vi "Y to D Conversion (Waveform).vi"(0 "phase voltage waveforms":waveform(dbl)[](array[waveform]), 9 "system info in":refnum<class "EP System Info.lvclass">, 11 "error in (no error)":errorcluster) -> (4 "line voltage waveforms":waveform(dbl)[](array[waveform]), 10 "system info out":refnum<class "EP System Info.lvclass">, 15 "error out":errorcluster)   [LabVIEW 2014, in "NI_EP_Power Quality.lvlib"]
doc: "Converts phase voltages to line voltages. You must manually select the polymorphic instance you want to use.\n\nThis VI supports measuring single-line and multiple-line systems."
uses:
  <vilib>/addons/Electrical Power/PQ/NI_EP_Power Quality.lvlib
  <vilib>/addons/Electrical Power/PQ/Common/Classes/System Info/EP System Info.lvclass
  <vilib>/addons/Electrical Power/Motor Monitoring/NI_EP_Motor Monitoring.lvlib
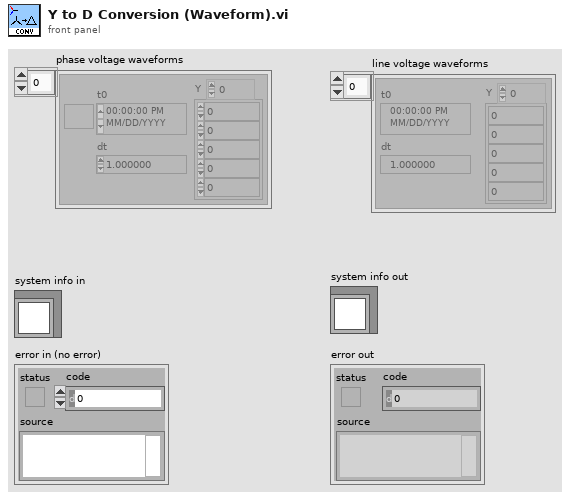
[diagram p1: front panel]
types:
  T1 = typedef "NI_EP_Power Quality.lvlib/ep_Wiring.ctl" = enum16{"4xUph + 4xI", "3xUph + 4xI", "3xUline + 4xI", "3xUph + 3xI", "3xUline + 3xI", "3xUph + 2xI", "3xUline + 2xI", "1xUph + 1xI"}
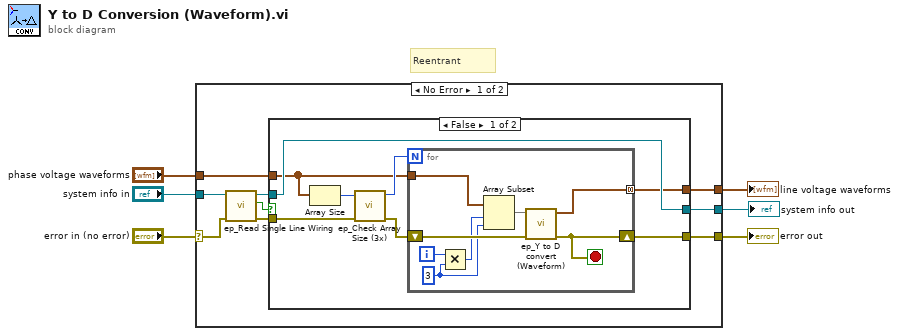
[diagram p0: block diagram]
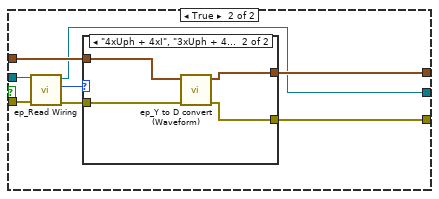
[diagram p2: hidden frame]
diagram:
  # "Reentrant"
  n1 = case shown="No Error" "error in (no error)" {
    selector: "error in (no error)" -> [w11 w48]
    tunnel: [w13 w48] -> w5
    tunnel: [w14 w47] -> w4
    tunnel: "phase voltage waveforms" -> [w15 w47]
    tunnel: "system info in" -> [w12 w46]
    tunnel: [w7 w46] -> w1
    frame No Error {
      n2 = call <vilib>:"ep_Read Single Line Wiring.vi"("error in (no error)"=w11, "system info in"=w12) -> ("error out"=w8:errorcluster, "single line wiring? (F)"=w10:bool, "system info out"=w9:refnum<class "EP System Info.lvclass">)  [unwired: 7 in]
      n3 = case shown="False" w10 {
        tunnel: w15 -> [w17 w36]
        tunnel: [w19 w34] -> w14
        tunnel: [w23 w33] -> w13
        tunnel: w9 -> [w22 w39]
        tunnel: w8 -> [w21 w38]
        tunnel: [w22 w32] -> w7
        frame False {
          n4 = Array Size(array=w17) -> (size(s)=w16:i32)
          n5 = call <vilib>:"ep_Check Array Size (3x).vi"("error in (no error)"=w21, "number of channels"=w16) -> ("error out"=w20:errorcluster, "number of 3 phases"=w18:i32)  [unwired: 8 in]
          n6 = for {
            N: w18 -> [_]
            shift-right: [w30] -> w23
            shift-left: w20 -> [w31]
            tunnel: [w29] -> w19 mode=concatenating
            tunnel: w17 -> [w28]
            i -> [w27]
            stop <- w30 stop-if-true
            w25 = 3 ("x")
            n7 = Multiply(x=w27, y=w25) -> (x*y=w26:i32)
            n8 = Array Subset(array=w28, index=w26, length=w25) -> (w24:waveform(dbl)[])
            n9 = call <vilib>:"ep_Y to D convert (Waveform).vi"("error in (no error)"=w31, "phase voltage waveforms"=w24) -> ("error out"=w30:errorcluster, "line voltage waveforms"=w29:waveform(dbl)[])  [unwired: 8 in]
          }
        }
        frame True {
          n10 = call <vilib>:"ep_Read Wiring.vi"("error in (no error)"=w38, "system info in"=w39) -> ("error out"=w35:errorcluster, "wiring"=w37:T1, "system info out"=w32:refnum<class "EP System Info.lvclass">)  [unwired: 6 in, 1 out]
          n11 = case shown="\"4xUph + 4xI\", \"3xUph + 4xI\", \"3xUph + 3xI\", \"3xUph + 2xI\"" w37 {
            tunnel: w36 -> [w41 w45]
            tunnel: w35 -> [w40 w44]
            tunnel: [w41 w43] -> w34
            tunnel: [w40 w42] -> w33
            frame Default {
            }
            frame "4xUph + 4xI", "3xUph + 4xI", "3xUph + 3xI", "3xUph + 2xI" {
              n12 = call <vilib>:"ep_Y to D convert (Waveform).vi"("error in (no error)"=w44, "phase voltage waveforms"=w45) -> ("error out"=w42:errorcluster, "line voltage waveforms"=w43:waveform(dbl)[])  [unwired: 8 in]
            }
          }
        }
      }
    }
    frame Error {
    }
  }
  "line voltage waveforms" <- w4
  "error out" <- w5
  "system info out" <- w1
